vi "Teleop.vi"(10 "Match Info":T1={"Autonomous Elapsed Seconds"=0.0, "TeleOp Elapsed Seconds"=0.0, "Disabled Elapsed Seconds"=0.0, "Visited Autonomous"=FALSE, "Visited TeleOp"=FALSE, "Visited Disabled"=FALSE, "Autonomous Settings"={"Autonomous Style"=enum."Independent", "VI Refnum"=refnum}}, 11 "Call Context":T2) -> ()   [LabVIEW 2017]
doc: "This VI is called for each enabled TeleOp packet received from the DS. It is typically used to read from joysticks and other inputs and update I/O or setpoints for timed control loops. It should complete and return within 20 milliseconds or risk missing DS packets."
uses:
  <vilib>/Rock Robotics/WPI/DriverStation/WPI_DriverStationDerivedRobotMode.ctl
  <vilib>/Rock Robotics/WPI/DriverStation/WPI_DriverStationMatch Info.ctl
  <vilib>/Rock Robotics/WPI/Utilities/WPI_GetSetVariantRefNum.vi
  <vilib>/Rock Robotics/Network Tables/NT Write Numeric Array.vi
  <vilib>/Rock Robotics/Network Tables/NT Write Boolean Array.vi
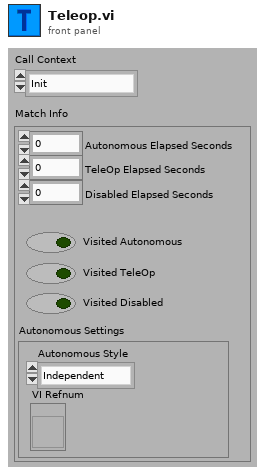
[diagram p1: front panel]
types:
  T1 = typedef "WPI_DriverStationMatch Info.ctl" = cluster{"Autonomous Elapsed Seconds":dbl, "TeleOp Elapsed Seconds":dbl, "Disabled Elapsed Seconds":dbl, "Visited Autonomous":bool, "Visited TeleOp":bool, "Visited Disabled":bool, "Autonomous Settings":cluster{"Autonomous Style":enum16{"Iterative", "Independent"}, "VI Refnum":refnum<vi>}}
  T2 = typedef "WPI_DriverStationDerivedRobotMode.ctl" = enum16{"Init", "Execute", "Stop"}
  T3 = typedef "WPI_JoystickDevRef.ctl" = cluster{"Device":T4}
  T4 = typedef "WPI_JoystickDeviceEnum.ctl" = enum16{"USB 0", "USB 1", "USB 2", "USB 3", "USB 4", "USB 5"}
  T5 = enum16{"Linear", "Square  Root", "Square", "n^x"}
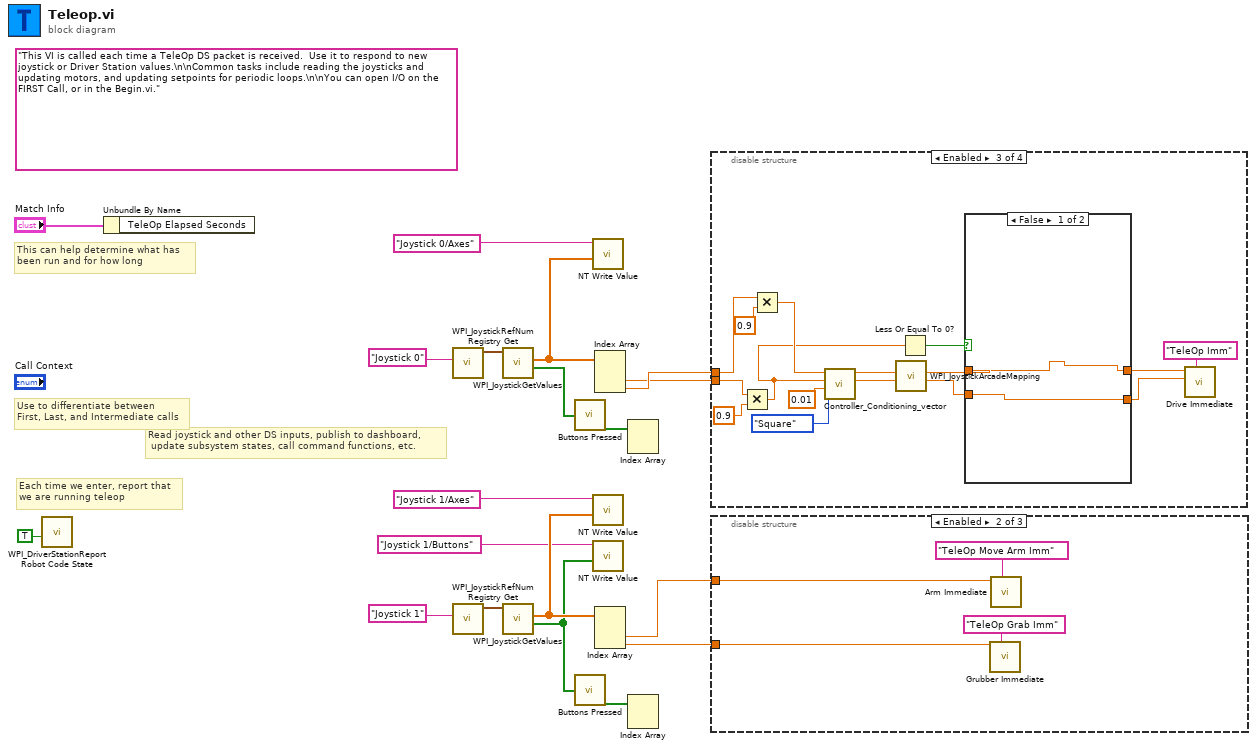
[diagram p0: block diagram]
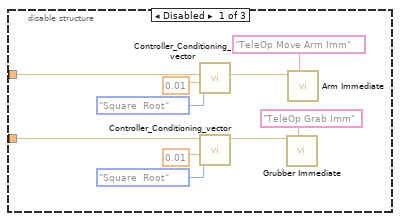
[diagram p2: hidden frame]
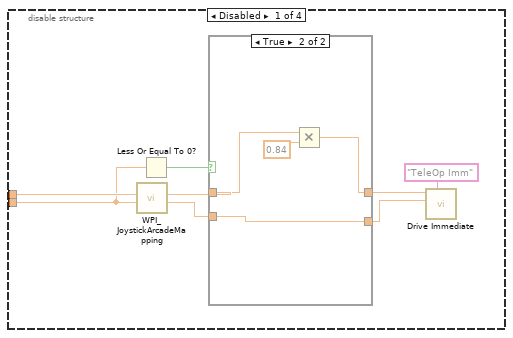
[diagram p4: hidden frame]
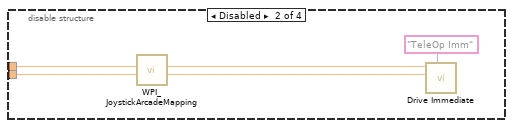
[diagram p6: hidden frame]
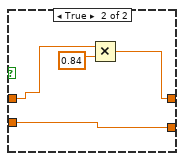
[diagram p7: hidden frame]
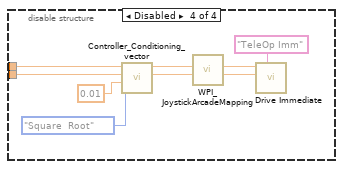
[diagram p8: hidden frame]
diagram:
  (unwired) "This VI is called each time a TeleOp DS packet is received.  Use it to respond to new joystick or Driver Station values.\n\nCommon tasks include reading the joysticks and updating motors, and updating setpoints for periodic loops.\n\nYou can open I/O on the FIRST Call, or in the Begin.vi."
  # "Read joystick and other DS inputs, publish to dashboard,\n update subsystem states, call command functions, etc."
  # "Each time we enter, report that\nwe are running teleop"
  # "Use to differentiate between\nFirst, Last, and Intermediate calls"
  # "This can help determine what has\nbeen run and for how long"
  n1 = call <vilib>:"WPI_DriverStationReport Robot Code State.vi"("TeleOp"=TRUE ("Autonomous")) -> ()  [unwired: 10 in, 1 out]
  n2 = Unbundle By Name("Match Info") -> ()  [unwired: 1 out]
  n3 = call <vilib>:"WPI_JoystickRefNum Registry Get.vi"("refnum name"="Joystick 0") -> ("JoystickDevRef"=w16:T3)  [unwired: 1 in, 9 out]
  n4 = call <vilib>:"WPI_JoystickRefNum Registry Get.vi"("refnum name"="Joystick 1") -> ("JoystickDevRef"=w5:T3)  [unwired: 1 in, 9 out]
  n5 = call <vilib>:"WPI_JoystickGetValues.vi"("JoystickDevRef"=w16) -> ("Buttons"=w14:bool[], "Axes"=w13:dbl[])  [unwired: 6 in, 3 out]
  n6 = call <vilib>:"WPI_JoystickGetValues.vi"("JoystickDevRef"=w5) -> ("Buttons"=w8:bool[], "Axes"=w9:dbl[])  [unwired: 6 in, 3 out]
  n7 = call "Buttons Pressed.vi"("Button Values"=w14) -> ("Button Presses"=w15:bool[])
  n8 = call "Buttons Pressed.vi"("Button Values"=w8) -> ("Button Presses"=w6:bool[])
  n9 = call-poly <vilib>:"NT Write Value.vi"("Numeric Array"=w13, "Name"="Joystick 0/Axes") -> ()  [unwired: 9 in, 1 out]
  n10 = call-poly <vilib>:"NT Write Value.vi"("Numeric Array"=w9, "Name"="Joystick 1/Axes") -> ()  [unwired: 9 in, 1 out]
  n11 = call-poly <vilib>:"NT Write Value.vi"("Boolean Array"=w8, "Name"="Joystick 1/Buttons") -> ()  [unwired: 9 in, 1 out]
  n12 = Index Array(array=w13) -> (element #2=w1:dbl, element #3=w11:dbl)  [unwired: 3 in, 1 out]
  n13 = Index Array(array=w9) -> (element #2=w3:dbl, element #3=w2:dbl)  [unwired: 3 in, 1 out]
  n14 = Index Array(array=w15) -> ()  [unwired: 2 in, 2 out]
  n15 = Index Array(array=w6) -> ()  [unwired: 2 in, 2 out]
  n16 = disable-structure shown="Enabled" {
    disable-tunnel: w11 -> [w26 w37 w44 w64]
    disable-tunnel: w1 -> [w20 w34 w40 w63]
    frame Disabled {
      n17 = call <vilib>:"WPI_JoystickArcadeMapping.vi"("Y axis value"=w20, "X axis value"=w26) -> ("Right Motor Value"=w23:dbl, "Left Motor Value"=w24:dbl)  [unwired: 8 in]
      n18 = Less Or Equal To 0?(x=w20) -> (x <= 0?=w25:bool)
      n19 = case shown="True" w25 {
        tunnel: w24 -> [w29 w31]
        tunnel: [w29 w30] -> w22
        tunnel: w23 -> [w28 w33]
        tunnel: [w28 w33] -> w21
        frame False {
        }
        frame True {
          n20 = Multiply(x=w31, y=0.84) -> (x*y=w30:dbl)
        }
      }
      n21 = call "Drive Immediate.vi"("Description"="TeleOp Imm", "Right Setpoint"=w21, "Left Setpoint"=w22) -> ()  [unwired: 8 in, 1 out]
    }
    frame Disabled {
      n22 = call <vilib>:"WPI_JoystickArcadeMapping.vi"("Y axis value"=w34, "X axis value"=w37) -> ("Right Motor Value"=w35:dbl, "Left Motor Value"=w36:dbl)  [unwired: 8 in]
      n23 = call "Drive Immediate.vi"("Description"="TeleOp Imm", "Right Setpoint"=w35, "Left Setpoint"=w36) -> ()  [unwired: 8 in, 1 out]
    }
    frame Enabled {
      n24 = Multiply(x=w40, y=0.9) -> (x*y=w39:dbl)
      n25 = Multiply(x=w44, y=0.9) -> (x*y=w42:dbl)
      n26 = call "Controller_Conditioning_vector.vi"("Enum"=T5."Square", "Dead Zone(0 to 1)"=0.01, "Y(-1 to 1)"=w39, "X(-1 to 1)"=w42) -> ("Y"=w45:dbl, "X"=w46:dbl)  [unwired: 4 in, 2 out]
      n27 = call <vilib>:"WPI_JoystickArcadeMapping.vi"("Y axis value"=w45, "X axis value"=w46) -> ("Right Motor Value"=w51:dbl, "Left Motor Value"=w52:dbl)  [unwired: 8 in]
      n28 = Less Or Equal To 0?(x=w39) -> (x <= 0?=w53:bool)
      n29 = case shown="False" w53 {
        tunnel: w52 -> [w55 w59]
        tunnel: [w55 w58] -> w50
        tunnel: w51 -> [w56 w57]
        tunnel: [w56 w57] -> w49
        frame False {
        }
        frame True {
          n30 = Multiply(x=w59, y=0.84) -> (x*y=w58:dbl)
        }
      }
      n31 = call "Drive Immediate.vi"("Description"="TeleOp Imm", "Right Setpoint"=w49, "Left Setpoint"=w50) -> ()  [unwired: 8 in, 1 out]
    }
    frame Disabled {
      n32 = call "Controller_Conditioning_vector.vi"("Enum"=T5."Square  Root", "Dead Zone(0 to 1)"=0.01, "Y(-1 to 1)"=w63, "X(-1 to 1)"=w64) -> ("Y"=w61:dbl, "X"=w62:dbl)  [unwired: 4 in, 2 out]
      n33 = call <vilib>:"WPI_JoystickArcadeMapping.vi"("Y axis value"=w61, "X axis value"=w62) -> ("Right Motor Value"=w67:dbl, "Left Motor Value"=w68:dbl)  [unwired: 8 in]
      n34 = call "Drive Immediate.vi"("Description"="TeleOp Imm", "Right Setpoint"=w67, "Left Setpoint"=w68) -> ()  [unwired: 8 in, 1 out]
    }
  }
  n35 = disable-structure shown="Enabled" {
    disable-tunnel: w3 -> [w74 w81 _]
    disable-tunnel: w2 -> [w73 w80 _]
    frame Disabled {
      n36 = call "Controller_Conditioning_vector.vi"("Enum"=T5."Square  Root", "Dead Zone(0 to 1)"=0.01, "Y(-1 to 1)"=w74) -> ("Y"=w77:dbl)  [unwired: 5 in, 3 out]
      n37 = call "Controller_Conditioning_vector.vi"("Enum"=T5."Square  Root", "Dead Zone(0 to 1)"=0.01, "X(-1 to 1)"=w73) -> ("X"=w72:dbl)  [unwired: 5 in, 3 out]
      n38 = call "Grubber Immediate.vi"("Description"="TeleOp Grab Imm", "Setpoint"=w72) -> ()  [unwired: 9 in, 1 out]
      n39 = call "Arm Immediate.vi"("Description"="TeleOp Move Arm Imm", "Setpoint"=w77) -> ()  [unwired: 9 in, 1 out]
    }
    frame Enabled {
      n40 = call "Grubber Immediate.vi"("Description"="TeleOp Grab Imm", "Setpoint"=w80) -> ()  [unwired: 9 in, 1 out]
      n41 = call "Arm Immediate.vi"("Description"="TeleOp Move Arm Imm", "Setpoint"=w81) -> ()  [unwired: 9 in, 1 out]
    }
    frame Disabled {
    }
  }
